vi "Database.ExportData.vi"(7 "Idx":i32, 8 "error in":errorcluster, 10 "Result in":T1, 11 "Data in":T6) -> (0 "error out":errorcluster, 1 "Export Time":timestamp, 2 "Result out":T1, 3 "Data out":T6)   [LabVIEW 2016]
doc: "Write test results (measurement values) to proda database\n\nWabco 2017 All right reserved\nAuthor: maciej.szupienko@wabco-auto.com"
uses:
  Database.Data.ctl
  Database.Data.Status.ctl
  Database.Data.Sets.ctl
  Cache/Cache.TestSteps.Fglb.ResultData.ctl
  ProdaNG/Controls/ProdaNG.ProcessResult.ctl
  ProdaNG/Controls/ProdaNG.ProcessStepResult.ctl
  ProdaNG/Controls/ProdaNG.TestStepResult.ctl
  ProdaNG/Controls/ProdaNG.TestValueResult.ctl
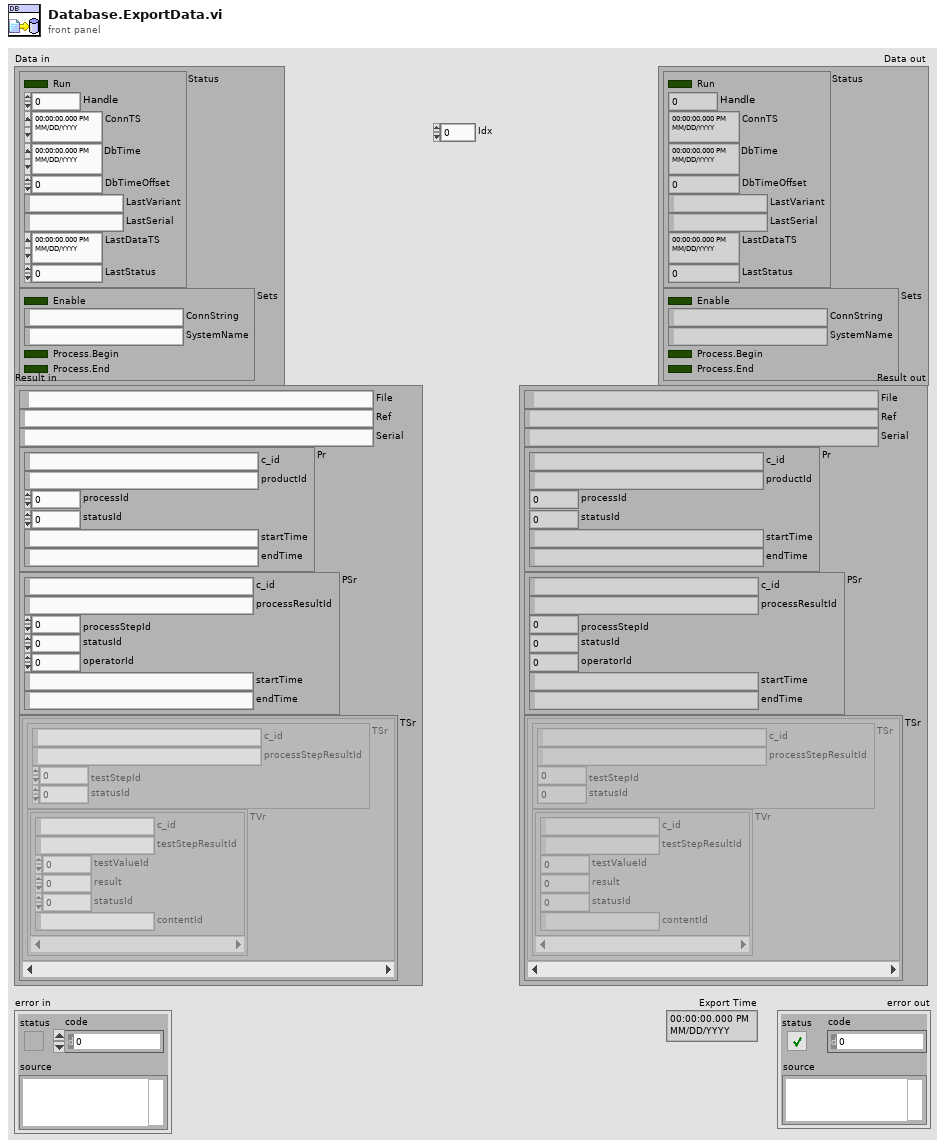
[diagram p1: front panel]
types:
  T1 = typedef "Cache.TestSteps.Fglb.ResultData.ctl" = cluster{"File":path, "Ref":string, "Serial":string, "Pr":T2, "PSr":T3, "TSr":cluster{"TSr":T4, "TVr":T5[]}[]}
  T2 = typedef "ProdaNG.ProcessResult.ctl" = cluster{"c_id":string, "productId":string, "processId":i32, "statusId":i32, "startTime":string, "endTime":string}
  T3 = typedef "ProdaNG.ProcessStepResult.ctl" = cluster{"c_id":string, "processResultId":string, "processStepId":i32, "statusId":i32, "operatorId":i32, "startTime":string, "endTime":string}
  T4 = typedef "ProdaNG.TestStepResult.ctl" = cluster{"c_id":string, "processStepResultId":string, "testStepId":i32, "statusId":i32}
  T5 = typedef "ProdaNG.TestValueResult.ctl" = cluster{"c_id":string, "testStepResultId":string, "testValueId":i32, "result":dbl, "statusId":i32, "contentId":string}
  T6 = typedef "Database.Data.ctl" = cluster{"Status":T7, "Sets":T8}
  T7 = typedef "Database.Data.Status.ctl" = cluster{"Run":bool, "Handle":i32, "ConnTS":timestamp, "DbTime":timestamp, "DbTimeOffset":dbl, "LastVariant":string, "LastSerial":string, "LastDataTS":timestamp, "LastStatus":i32}
  T8 = typedef "Database.Data.Sets.ctl" = cluster{"Enable":bool, "ConnString":string, "SystemName":string, "Process.Begin":bool, "Process.End":bool}
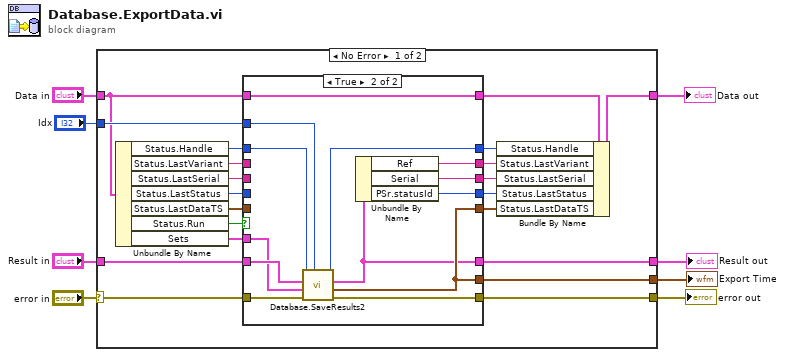
[diagram p0: block diagram]
diagram:
  n1 = case shown="No Error" "error in" {
    selector: "error in" -> [w25 w51]
    tunnel: [w26 w51] -> w8
    tunnel: "Data in" -> [w10 w50]
    tunnel: [w27 w50] -> w5
    tunnel: "Result in" -> [w21 _]
    tunnel: [w24 _] -> w3
    tunnel: [w22 _] -> w2
    tunnel: "Idx" -> [w11 _]
    frame No Error {
      n2 = Unbundle By Name(w10) -> ("Status.Handle"=w29:i32, "Status.LastVariant"=w18:string, "Status.LastSerial"=w17:string, "Status.LastStatus"=w15:i32, "Status.LastDataTS"=w13:timestamp, "Status.Run"=w23:bool, "Sets"=w14:T8)
      n3 = case shown="True" w23 {
        tunnel: w29 -> [w35 w49]
        tunnel: [w35 w38] -> w28
        tunnel: [w36 w43] -> w26
        tunnel: w25 -> [w36 w48]
        tunnel: w21 -> [_ w44]
        tunnel: [_ w37] -> w24
        tunnel: [_ w42] -> w22
        tunnel: [w34 w47] -> w20
        tunnel: [w33 w46] -> w19
        tunnel: w18 -> [w34 _]
        tunnel: w17 -> [w33 _]
        tunnel: [w32 w45] -> w16
        tunnel: w15 -> [w32 _]
        tunnel: w14 -> [_ w39]
        tunnel: w13 -> [w31 _]
        tunnel: [w31 w42] -> w12
        tunnel: w11 -> [_ w40]
        tunnel: w10 -> [w30 w41]
        tunnel: [w30 w41] -> w9
        frame False {
        }
        frame True {
          n4 = call "Database.SaveResults2.vi"("Idx"=w40, "error in (no error)"=w48, "Sets"=w39, "Data to export"=w44, "dbHandle"=w49) -> ("error out"=w43:errorcluster, "Export Time"=w42:timestamp, "Data exported"=w37:T1, "dbHandle out"=w38:i32)  [unwired: 3 in]
          n5 = Unbundle By Name(w37) -> ("Ref"=w47:string, "Serial"=w46:string, "PSr.statusId"=w45:i32)
        }
      }
      n6 = Bundle By Name(cluster=w9, "Status.Handle"=w28, "Status.LastVariant"=w20, "Status.LastSerial"=w19, "Status.LastStatus"=w16, "Status.LastDataTS"=w12) -> (w27:T6)
    }
    frame Error {
    }
  }
  "error out" <- w8
  "Data out" <- w5
  "Result out" <- w3
  "Export Time" <- w2
